vi "CRYMeasured Fre-SPL.vi"() -> (6 "measured frequency":dbl[](array[numeric]), 8 "measured SPL":dbl[](array[numeric]))   [LabVIEW 2013]
panel:
  out "XY Graph":cluster{"XY Graph":cluster{dbl, dbl}[]}[](graph)
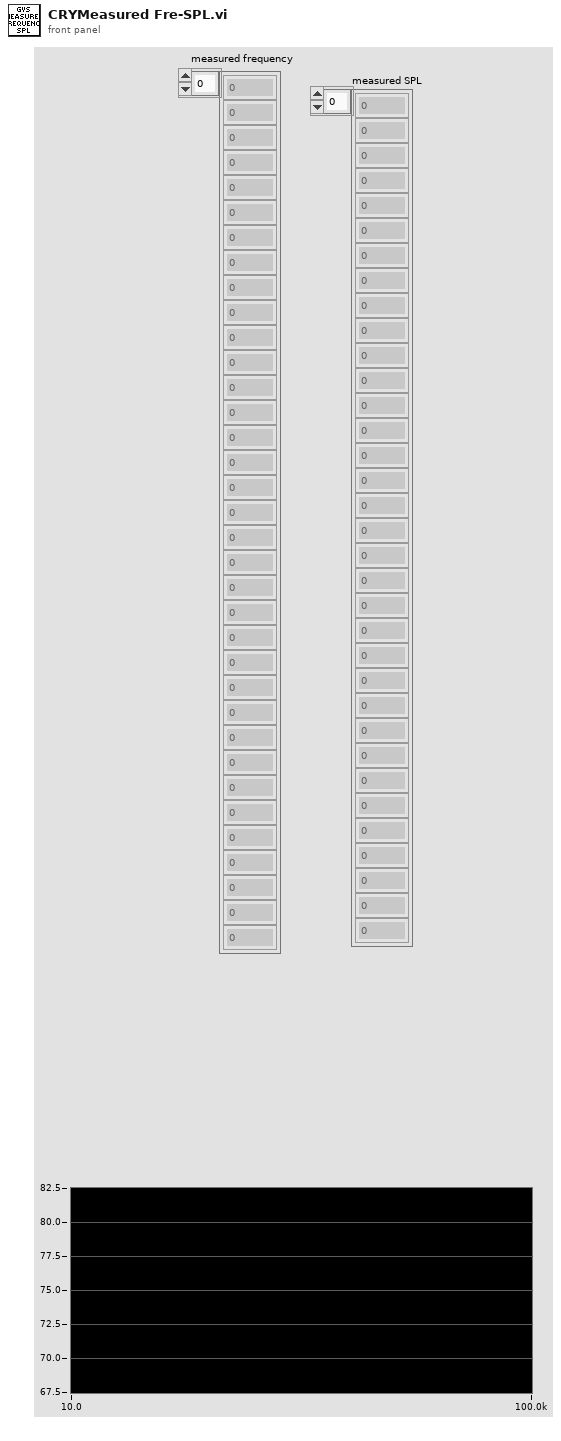
[diagram p1: front panel]
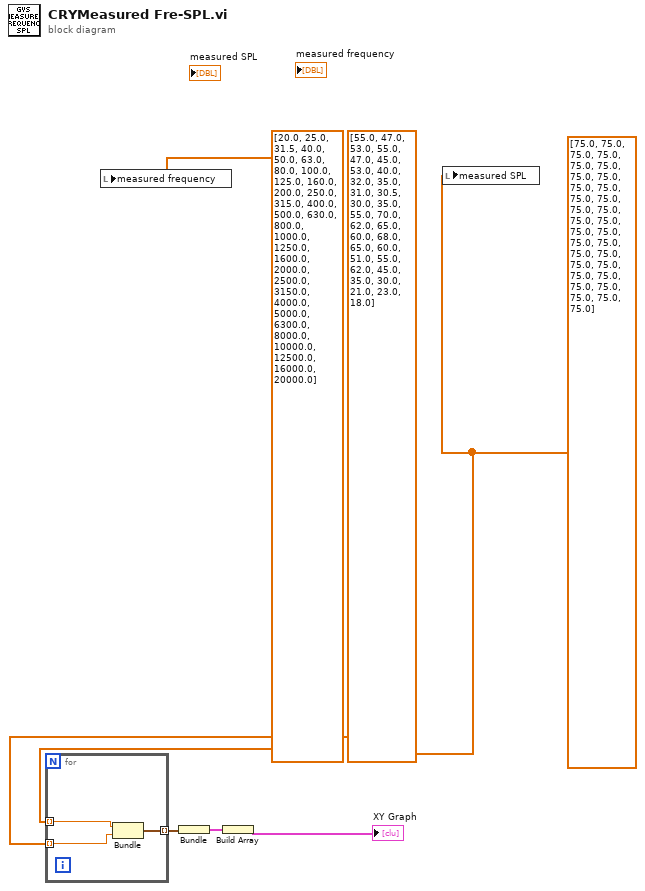
[diagram p0: block diagram]
diagram:
  w1 = dbl[] [75.0, 75.0, 75.0, 75.0, 75.0, 75.0, 75.0, 75.0, 75.0, 75.0, 75.0, 75.0, 75.0, 75.0, 75.0, 75.0, 75.0, 75.0, 75.0, 75.0, 75.0, 75.0, 75.0, 75.0, 75.0, 75.0, 75.0, 75.0, 75.0, 75.0, 75.0]
  w2 = dbl[] [20.0, 25.0, 31.5, 40.0, 50.0, 63.0, 80.0, 100.0, 125.0, 160.0, 200.0, 250.0, 315.0, 400.0, 500.0, 630.0, 800.0, 1000.0, 1250.0, 1600.0, 2000.0, 2500.0, 3150.0, 4000.0, 5000.0, 6300.0, 8000.0, 10000.0, 12500.0, 16000.0, 20000.0]
  (unwired) dbl[] [55.0, 47.0, 53.0, 55.0, 47.0, 45.0, 53.0, 40.0, 32.0, 35.0, 31.0, 30.5, 30.0, 35.0, 55.0, 70.0, 62.0, 65.0, 60.0, 68.0, 65.0, 60.0, 51.0, 55.0, 62.0, 45.0, 35.0, 30.0, 21.0, 23.0, 18.0]
  n1 = for {
    tunnel: [w8] -> w3 mode=indexing
    tunnel: w2 -> [w7] mode=indexing
    tunnel: w1 -> [w6] mode=indexing
    n2 = Bundle(w7, w6) -> (w8:cluster{dbl, dbl})  [unwired: 1 out]
  }
  n3 = local write "measured frequency"(w2) -> ()
  n4 = Bundle(w3) -> (w5:cluster{cluster{dbl, dbl}[]})  [unwired: 1 in]
  n5 = Build Array(w5) -> (→"XY Graph":cluster{cluster{dbl, dbl}[]}[])
  n6 = local write "measured SPL"(w1) -> ()
